vi "HackRF_Close.vi"(8 "error in (no error)":errorcluster, 11 "Cluster in":T1) -> (0 "error out":errorcluster, 3 "Cluster out":T1)   [LabVIEW 2021]
uses:
  HackRF_Ref.ctl
  C:/Program Files/HackRF/labview/x64/NetHackrfx64.dll
  NetHackrfx64.dll
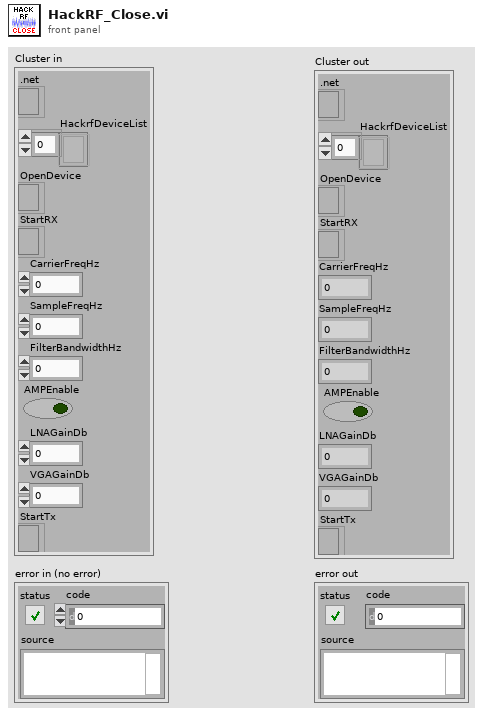
[diagram p1: front panel]
types:
  T1 = typedef "HackRF_Ref.ctl" = cluster{".net":refnum<k24>, "HackrfDeviceList":refnum<k24>[], "OpenDevice":refnum<k24>, "StartRX":refnum<k24>, "CarrierFreqHz":dbl, "SampleFreqHz":dbl, "FilterBandwidthHz":dbl, "AMPEnable":bool, "LNAGainDb":dbl, "VGAGainDb":dbl, "StartTx":refnum<k24>}
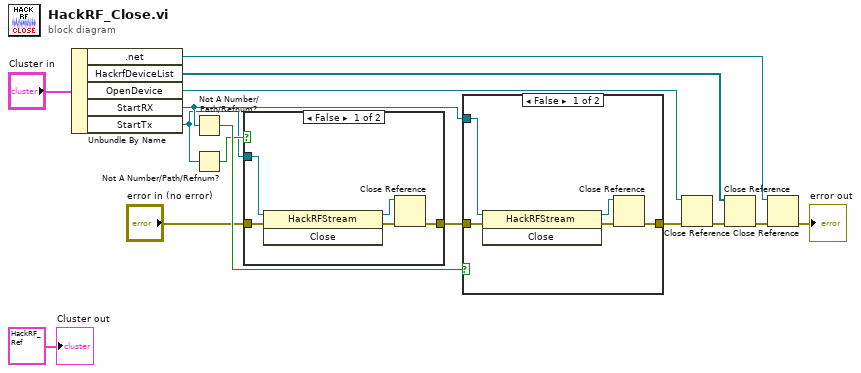
[diagram p0: block diagram]
diagram:
  n1 = Unbundle By Name("Cluster in") -> (".net"=w6:refnum<k24>, "HackrfDeviceList"=w8:refnum<k24>[], "OpenDevice"=w10:refnum<k24>, "StartRX"=w12:refnum<k24>, "StartTx"=w1:refnum<k24>)
  n2 = Not A Number/Path/Refnum?(number/path/refnum=w12) -> (NaN/Path/Refnum?=w13:bool)
  n3 = Not A Number/Path/Refnum?(number/path/refnum=w1) -> (NaN/Path/Refnum?=w4:bool)
  n4 = case shown="False" w4 {
    tunnel: "error in (no error)" -> [w20 w21]
    tunnel: w1 -> [w19 _]
    tunnel: [w16 w21] -> w3
    frame False {
      n5 = invoke class="HackRFStream" method="Close"(reference=w19, error in=w20) -> (reference out=w17:refnum<k24>, error out=w18:errorcluster)  [unwired: 1 in, 1 out]
      n6 = Close Reference(reference=w17, error in (no error)=w18) -> (error out=w16:errorcluster)
    }
    frame True {
    }
  }
  n7 = case shown="False" w13 {
    tunnel: w3 -> [w26 w27]
    tunnel: w12 -> [w25 _]
    tunnel: [w22 w27] -> w11
    frame False {
      n8 = invoke class="HackRFStream" method="Close"(reference=w25, error in=w26) -> (reference out=w23:refnum<k24>, error out=w24:errorcluster)  [unwired: 1 in, 1 out]
      n9 = Close Reference(reference=w23, error in (no error)=w24) -> (error out=w22:errorcluster)
    }
    frame True {
    }
  }
  n10 = Close Reference(reference=w10, error in (no error)=w11) -> (error out=w9:errorcluster)
  n11 = Close Reference(reference=w8, error in (no error)=w9) -> (error out=w7:errorcluster)
  n12 = Close Reference(reference=w6, error in (no error)=w7) -> (error out=→"error out":errorcluster)
  "Cluster out" <- T1 {".net"=refnum, "HackrfDeviceList"=[], "OpenDevice"=refnum, "StartRX"=refnum, "CarrierFreqHz"=0.0, "SampleFreqHz"=0.0, "FilterBandwidthHz"=0.0, "AMPEnable"=FALSE, "LNAGainDb"=0.0, "VGAGainDb"=0.0, "StartTx"=refnum} ("Cluster")
